vi "XYZ Stage-Cleanup.vi"(8 "error in (no error)":errorcluster, 11 "XY Stage config cluster":T1={"COM port"="COM7", "XY stage available"=FALSE}) -> (0 "error out":errorcluster)   [LabVIEW 2013]
uses:
  Typedefs/XY Stage config cluster.ctl
  <vilib>/Utility/error.llb/DialogType.ctl
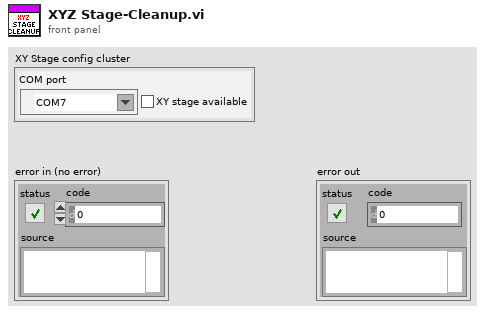
[diagram p1: front panel]
types:
  T1 = typedef "XY Stage config cluster.ctl" = cluster{"COM port":refnum<visa-resource-name>, "XY stage available":bool}
  T2 = typedef "DialogType.ctl" = u16
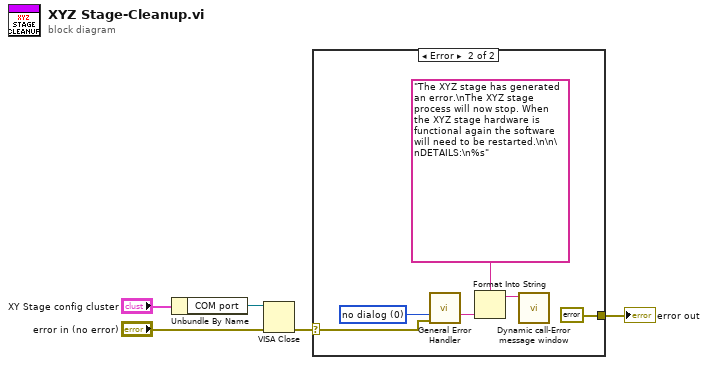
[diagram p0: block diagram]
diagram:
  n1 = Unbundle By Name("XY Stage config cluster") -> ("COM port"=w4:refnum<visa-resource-name>)
  n2 = VISA Close(VISA resource name=w4, error in (no error)="error in (no error)") -> (error out=w5:errorcluster)
  n3 = case shown="Error" w5 {
    selector: w5 -> [_ w7]
    tunnel: [_ errorcluster {"status"=FALSE, "code"=0, "source"=""} ("error out")] -> w2
    frame No Error {
    }
    frame Error {
      w9 = T2 0 items=["no dialog", "OK message", "continue or stop message", "OK message + warnings", "continue/stop + warnings"] ("type of dialog (OK msg:1)")
      n4 = call <vilib>:"General Error Handler.vi"("type of dialog (OK msg:1)"=w9, "error in (no error)"=w7) -> ("message"=w8:string)  [unwired: 9 in, 4 out]
      n5 = Format Into String(format string="The XYZ stage has generated an error.\nThe XYZ stage process will now stop. When the XYZ stage hardware is functional again the software will need to be restarted.\n\n\nDETAILS:\n%s" ("Error Source"), w8) -> (resulting string=w6:string)  [unwired: 2 in, 1 out]
      n6 = call "Dynamic call-Error message window.vi"("Error Message"=w6) -> ()  [unwired: 10 in, 1 out]
    }
  }
  "error out" <- w2
